vi "finishUp.vi"(8 "error in (no error)":errorcluster, 11 "StaticOutputEditor in":refnum<class "StaticOutputEditor.lvclass">) -> (0 "error out":errorcluster, 3 "StaticOutputEditor out":refnum<class "StaticOutputEditor.lvclass">)   [LabVIEW 2009, in "Views.lvlib" / "ScriptEditor.lvlib" / "StaticOutputEditor.lvclass"]
uses:
  StaticOutputEditor.lvclass
  StaticOutputEditor.lvclass/StaticOutputEditor.ctl
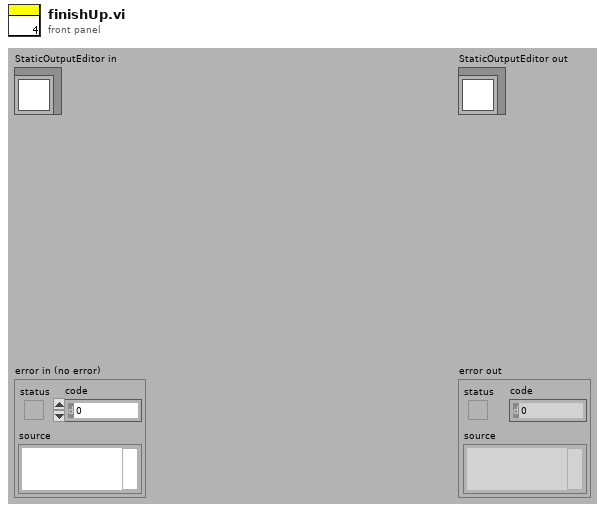
[diagram p1: front panel]
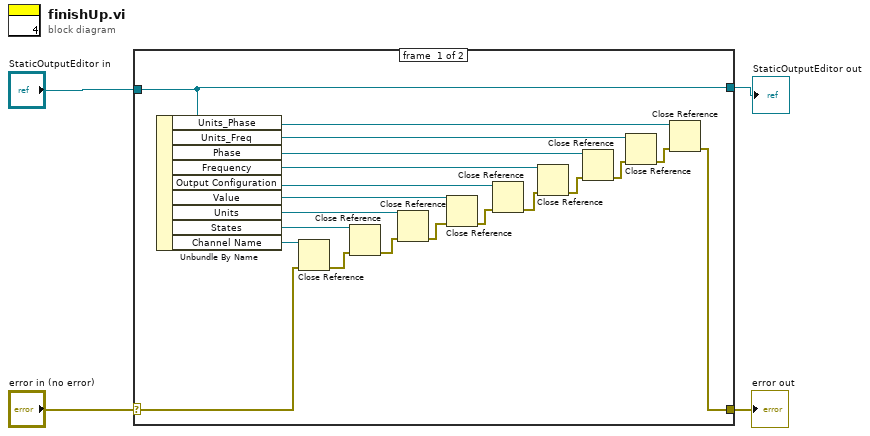
[diagram p0: block diagram]
diagram:
  n1 = case shown="No Error" "error in (no error)" {
    selector: "error in (no error)" -> [w16 w26]
    tunnel: [w5 w26] -> w3
    tunnel: [w24 w25] -> w1
    tunnel: "StaticOutputEditor in" -> [w24 w25]
    frame #0 {
      n2 = Unbundle By Name(w24) -> ("Units_Phase"=w10:refnum<vi>, "Units_Freq"=w11:refnum<vi>, "Phase"=w12:refnum<vi>, "Frequency"=w13:refnum<vi>, "Output Configuration"=w15:refnum<vi>, "Value"=w23:refnum<vi>, "Units"=w22:refnum<vi>, "States"=w21:refnum<vi>, "Channel Name"=w20:refnum<vi>)
      n3 = Close Reference(reference=w20, error in (no error)=w16) -> (error out=w17:errorcluster)
      n4 = Close Reference(reference=w21, error in (no error)=w17) -> (error out=w18:errorcluster)
      n5 = Close Reference(reference=w22, error in (no error)=w18) -> (error out=w19:errorcluster)
      n6 = Close Reference(reference=w23, error in (no error)=w19) -> (error out=w14:errorcluster)
      n7 = Close Reference(reference=w15, error in (no error)=w14) -> (error out=w6:errorcluster)
      n8 = Close Reference(reference=w13, error in (no error)=w6) -> (error out=w9:errorcluster)
      n9 = Close Reference(reference=w12, error in (no error)=w9) -> (error out=w8:errorcluster)
      n10 = Close Reference(reference=w11, error in (no error)=w8) -> (error out=w7:errorcluster)
      n11 = Close Reference(reference=w10, error in (no error)=w7) -> (error out=w5:errorcluster)
    }
    frame #1 {
    }
  }
  "error out" <- w3
  "StaticOutputEditor out" <- w1
